vi "7.1 Auto Act Loop.vi"() -> ()   [LabVIEW 2010]
uses:
  4-High Neurons/4.0-Timing Badass.ctl
  6-OCU Neurons/6.1-Act.ctl
  6-OCU Neurons/6.1-UDP Saitek.ctl
  <vilib>/Utility/inputDevices.llb/closeJoystick.vi
  7.0-Global.vi
  <vilib>/Utility/inputDevices.llb/joystickAcquire.vi
panel:
  in  "Stop":bool
  out "output cluster":T1 {"6.1-Saitek Controller"."Right" scale=-32767.0..32767.0; "6.1-Saitek Controller"."Left" scale=-32767.0..32767.0; "6.1-Saitek Controller"."Yaw" scale=-32767.0..32767.0; "6.1-Saitek Controller"."Roll" scale=-32767.0..32767.0; "6.1-Saitek Controller"."Pitch" scale=-32767.0..32767.0}
  out "Super Heart Beat":T3
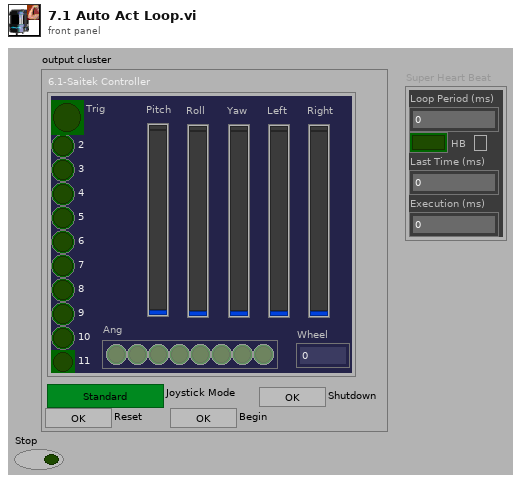
[diagram p1: front panel]
types:
  T1 = typedef "6.1-Act.ctl" = cluster{"6.1-Saitek Controller":T2, "Joystick Mode":bool, "Shutdown":bool, "Reset":bool, "Begin":bool}
  T2 = typedef "6.1-UDP Saitek.ctl" = cluster{"Trig":bool, "2":bool, "3":bool, "4":bool, "5":bool, "6":bool, "7":bool, "8":bool, "9":bool, "10":bool, "11":bool, "Pitch":i32, "Ang":bool[], "Wheel":dbl, "Roll":i32, "Yaw":i32, "Left":i32, "Right":i32}
  T3 = typedef "4.0-Timing Badass.ctl" = cluster{"Loop Period (ms)":u32, "HB":bool, "Last Time (ms)":u32, "Execution (ms)":u32}
  T4 = typedef "7.0 Auto Mode Buttons.ctl" = cluster{"Enable Joystick":bool, "End Run":bool, "Begin":bool, "Send Map":bool}
  T5 = cluster{"X axis":i32, "Y axis":i32, "Z axis":i32, "X axis rotation":i32, "Y axis rotation":i32, "Z axis rotation":i32, "U axis":i32, "V axis":i32}
  T6 = cluster{"button 1":bool, "button 2":bool, "button 3":bool, "button 4":bool, "button 5":bool, "button 6":bool, "button 7":bool, "button 8":bool, "button 9":bool, "button 10":bool, "button 11":bool, "button 12":bool, "button 13":bool, "button 14":bool, "button 15":bool, "button 16":bool, "button 17":bool, "button 18":bool, "button 19":bool, "button 20":bool, "button 21":bool, "button 22":bool, "button 23":bool, "button 24":bool, "button 25":bool, "button 26":bool, "button 27":bool, "button 28":bool, "button 29":bool, "button 30":bool, "button 31":bool, "button 32":bool}
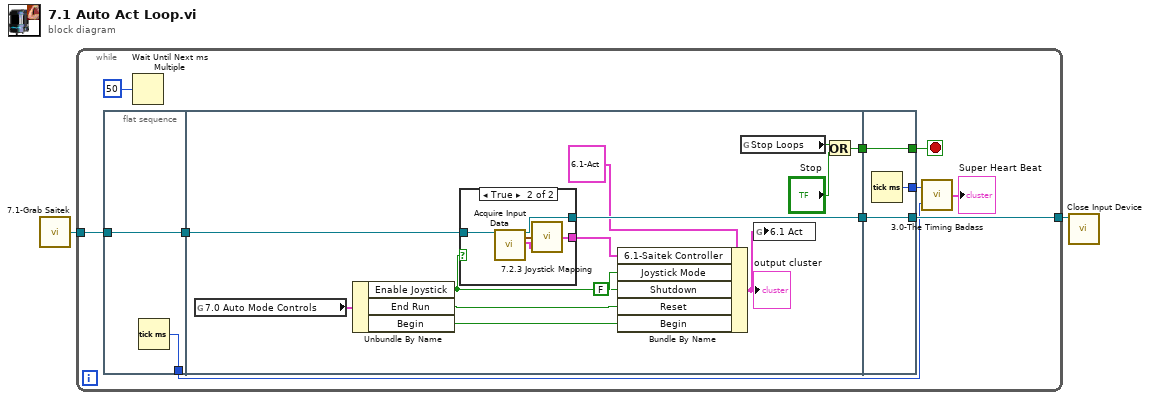
[diagram p0: block diagram]
diagram:
  n1 = call "7.1-Grab Saitek.vi"() -> ("Saitek ID"=w1:refnum<k1>)
  n2 = while {
    tunnel: w1 -> [w11]
    tunnel: [w10] -> w2
    stop <- w12 stop-if-true
    n3 = flat-sequence {
      tunnel: w11 -> [w14]
      tunnel: [w14] -> w7
      tunnel: [w13] -> w5
      tunnel: [w18] -> w9
      tunnel: [w25] -> w8
      tunnel: w7 -> [w26]
      tunnel: [w35] -> w10
      tunnel: [w36] -> w12
      tunnel: w9 -> [w36]
      tunnel: w8 -> [w35]
      tunnel: [w34] -> w6
      frame #0 {
        n4 = Tick Count (ms)() -> (millisecond timer value=w13:u32)
      }
      frame #1 {
        n5 = global read "7.0-Global.vi" "7.0 Auto Mode Controls"() -> (w21:T4)
        n6 = Unbundle By Name(w21) -> ("Enable Joystick"=w16:bool, "End Run"=w20:bool, "Begin"=w19:bool)
        n7 = case shown="True" w16 {
          tunnel: w26 -> [w28 w33]
          tunnel: [w28 w30] -> w25
          tunnel: [_ w29] -> w22
          frame False {
          }
          frame True {
            n8 = call-poly <vilib>:"Acquire Input Data.vi"("device ID"=w33) -> ("device ID"=w30:refnum<k1>, "axis info"=w32:T5, "button info"=w31:T6)  [unwired: 14 in, 2 out]
            n9 = call "7.2.3 Joystick Mapping.vi"("button info"=w31, "axis info"=w32) -> ("Joystick Out"=w29:T2)  [unwired: 1 in]
          }
        }
        n10 = Bundle By Name(cluster=T1 {"6.1-Saitek Controller"={"Trig"=FALSE, "2"=FALSE, "3"=FALSE, "4"=FALSE, "5"=FALSE, "6"=FALSE, "7"=FALSE, "8"=FALSE, "9"=FALSE, "10"=FALSE, "11"=FALSE, "Pitch"=0, "Ang"=[], "Wheel"=0.0, "Roll"=0, "Yaw"=0, "Left"=0, "Right"=0}, "Joystick Mode"=FALSE, "Shutdown"=FALSE, "Reset"=FALSE, "Begin"=FALSE} ("6.1 Act"), "6.1-Saitek Controller"=w22, "Joystick Mode"=w16, "Shutdown"=FALSE, "Reset"=w20, "Begin"=w19) -> (w23:T1)
        "output cluster" <- w23
        n11 = global read "7.0-Global.vi" "Stop Loops"() -> (w27:bool)
        n12 = global write "7.0-Global.vi" "6.1 Act"(w23) -> ()
        n13 = Or(x=w27, y="Stop") -> (x .or. y?=w18:bool)
      }
      frame #2 {
        n14 = Tick Count (ms)() -> (millisecond timer value=w34:u32)
      }
    }
    n15 = Wait Until Next ms Multiple(millisecond multiple=u32 50) -> ()  [unwired: 1 out]
    n16 = call "3.0-The Timing Badass.vi"("Start"=w5, "End"=w6) -> ("Super Heart Beat"=→"Super Heart Beat":T3)
  }
  n17 = call-poly <vilib>:"Close Input Device.vi"("device ID"=w2) -> ()  [unwired: 9 in, 1 out]
